vi "battery-sim-exec.vi"(10 "Nominal Battery\nVoltage":dbl, 11 "Current Amps":dbl) -> (3 "Loaded Voltage":dbl)   [LabVIEW 2019]
uses:
  <vilib>/Rock Robotics/WPI/ThirdParty/JAS_Junk/TrajLib/Trajectory_Library.lvlib
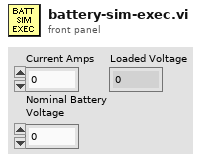
[diagram p1: front panel]
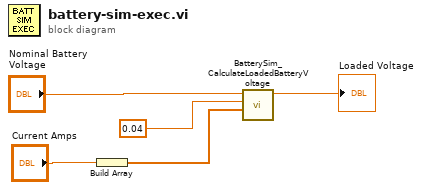
[diagram p0: block diagram]
diagram:
  n1 = Build Array("Current Amps") -> (w1:dbl[])
  n2 = call <vilib>:"BatterySim_CalculateLoadedBatteryVoltage.vi"("Currents"=w1, "Resistance_Ohms"=0.04, "NominalVoltage"="Nominal Battery\nVoltage") -> ("Voltage"=→"Loaded Voltage":dbl)  [unwired: 8 in]
